vi "Main.vi"() -> ()   [LabVIEW 2016]
uses:
  Experiment States.ctl
  <vilib>/DAQmx/read.llb/DAQmx Read (Analog 2D DBL NChan NSamp).vi
  <vilib>/DAQmx/miscellaneous.llb/DAQmx Fill In Error Info.vi
panel:
  out "T1 12":dbl
  out "T1 11":dbl
  out "T1 10":dbl
  out "T1 9":dbl
  out "T1 8":dbl
  out "T1 7":dbl
  out "T1 6":dbl
  out "T1 5":dbl
  out "T1 4":dbl
  out "T1 3":dbl
  out "T1 2":dbl
  out "T1":dbl
  out "Thermocouple 12":cluster{"X":dbl, "Y":dbl}[](graph)
  out "Thermocouple 11":cluster{"X":dbl, "Y":dbl}[](graph)
  out "Thermocouple 10":cluster{"X":dbl, "Y":dbl}[](graph)
  out "Thermocouple 9":cluster{"X":dbl, "Y":dbl}[](graph)
  out "Thermocouple 8":cluster{"X":dbl, "Y":dbl}[](graph)
  out "Thermocouple 7":cluster{"X":dbl, "Y":dbl}[](graph)
  out "Thermocouple 6":cluster{"X":dbl, "Y":dbl}[](graph)
  out "Thermocouple 5":cluster{"X":dbl, "Y":dbl}[](graph)
  out "Thermocouple 4":cluster{"X":dbl, "Y":dbl}[](graph)
  out "Thermocouple 3":cluster{"X":dbl, "Y":dbl}[](graph)
  out "Thermocouple 2":cluster{"X":dbl, "Y":dbl}[](graph)
  out "Thermocouple 1":cluster{"X":dbl, "Y":dbl}[](graph)
  in  "Thermocouple 12 Channel":tag
  in  "Thermocouple 11 Channel":tag
  in  "Thermocouple 10 Channel":tag
  in  "Thermocouple 9 Channel":tag
  in  "Thermocouple 8 Channel":tag
  in  "Thermocouple 7 Channel":tag
  in  "Thermocouple 6 Channel":tag
  in  "Thermocouple 5 Channel":tag
  in  "Thermocouple 4 Channel":tag
  in  "Thermocouple 3 Channel":tag
  in  "Thermocouple 2 Channel":tag
  in  "Thermocouple 1 Channel":tag
  in  "End Experiment?":bool
  in  "Start":bool
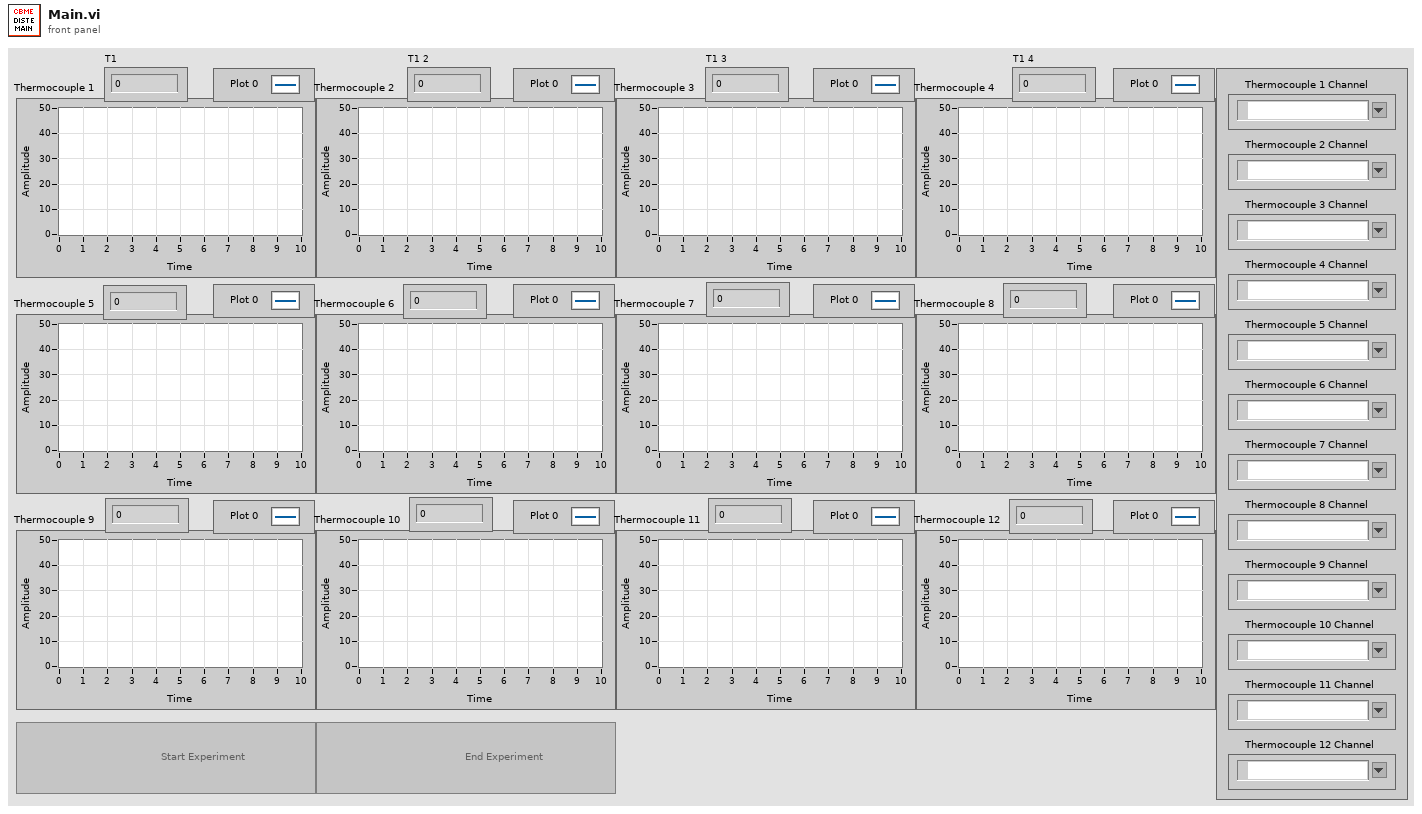
[diagram p1: front panel]
types:
  T1 = typedef "Experiment States.ctl" = enum16{"Setup", "Data Collection", "Export", "Finish"}
  T2 = enum8{"Enabled", "Disabled", "Disabled and Grayed Out"}
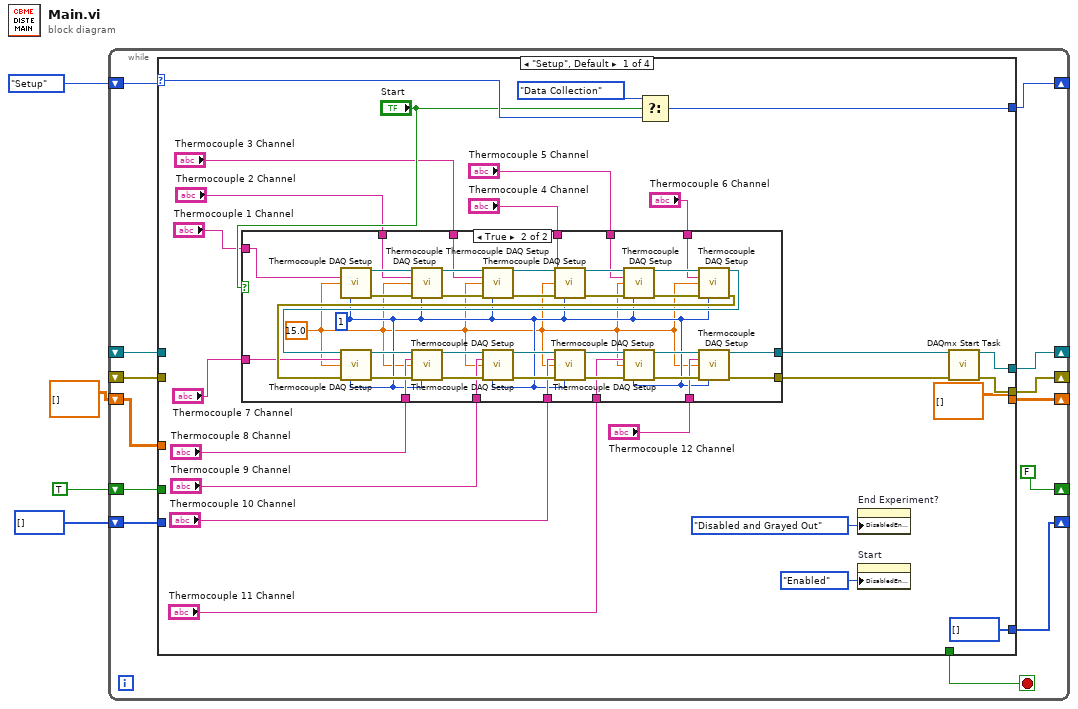
[diagram p0: block diagram]
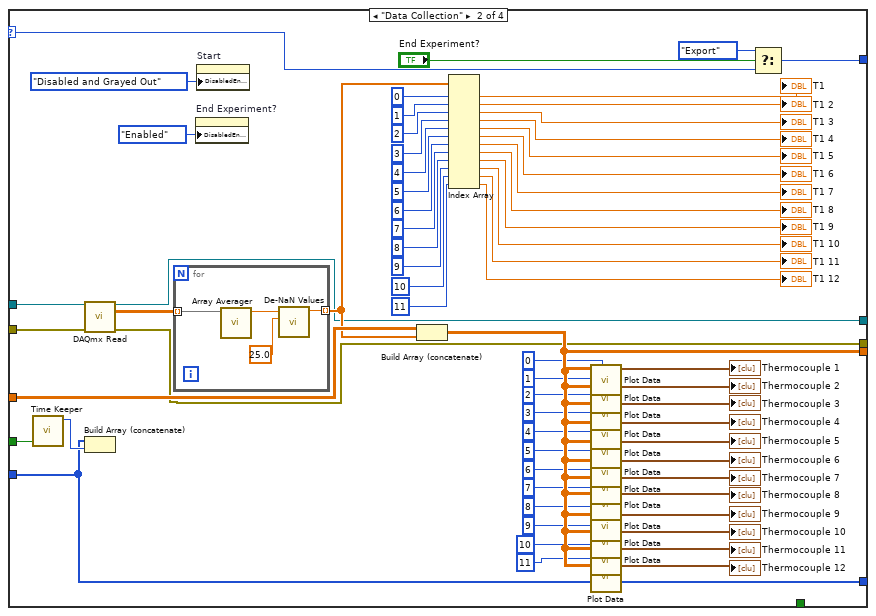
[diagram p3: hidden frame]
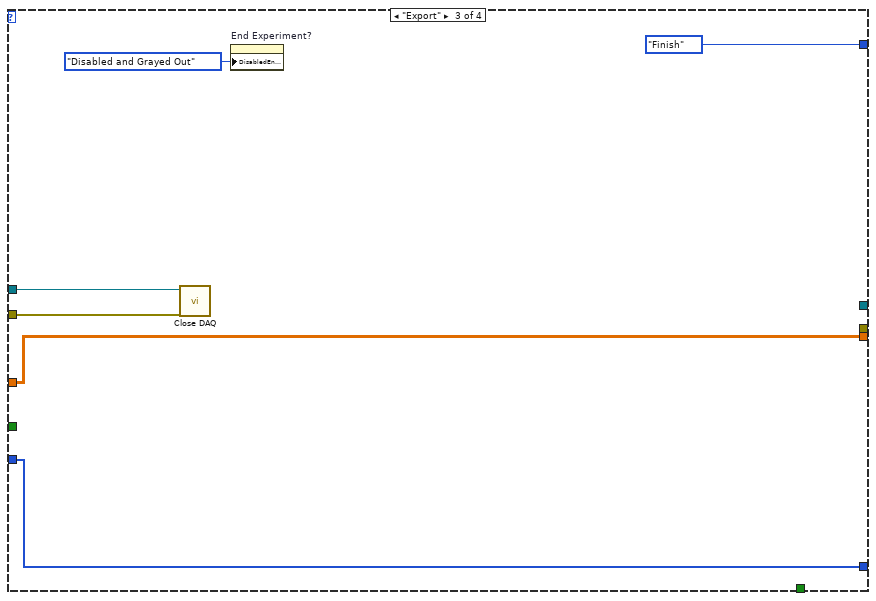
[diagram p4: hidden frame]
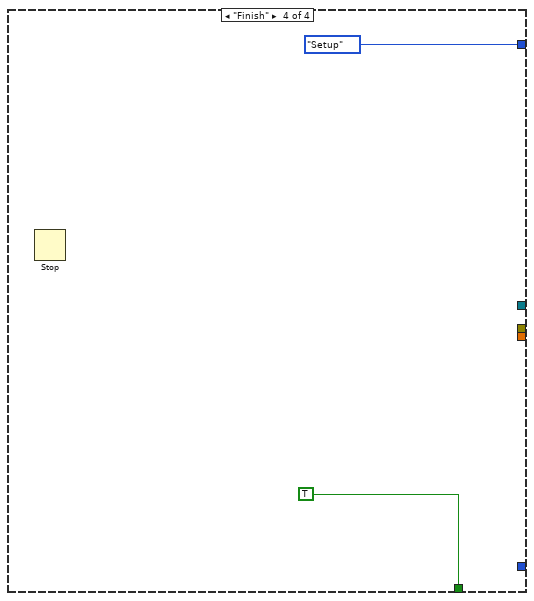
[diagram p5: hidden frame]
diagram:
  n1 = while {
    shift-right: [w16] -> _
    shift-left: Experiment_States."Setup" ("Enum") -> [w17]
    shift-right: [w13] -> _
    shift-left: _ -> [w11]
    shift-right: [w14] -> _
    shift-left: _ -> [w12]
    shift-right: [w10] -> _
    shift-left: dbl[][] [] -> [w9]
    shift-right: [FALSE ("Reset?")] -> _
    shift-left: TRUE ("Reset?") -> [w8]
    shift-right: [w5] -> _
    shift-left: u32[] [] -> [w7]
    stop <- w15 stop-if-true
    n2 = case shown="\"Setup\", Default" w17 {
      selector: w17 -> [w41 w142 _ _]
      tunnel: [w39 w144 Experiment_States."Finish" ("Enum") Experiment_States."Setup" ("Enum")] -> w16
      tunnel: [_ _ _ TRUE] -> w15
      tunnel: [w24 w81 _ _] -> w14
      tunnel: [w22 w80 _ _] -> w13
      tunnel: w12 -> [_ w140 w151 _]
      tunnel: w11 -> [_ w139 w150 _]
      tunnel: [dbl[][] [] w97 w152 _] -> w10
      tunnel: w9 -> [_ w113 w152 _]
      tunnel: w8 -> [_ w110 _ _]
      tunnel: w7 -> [_ w84 w153 _]
      tunnel: [u32[] [] w84 w153 _] -> w5
      frame "Setup", Default {
        n3 = case shown="True" "Start" {
          tunnel: [_ w57] -> w38
          tunnel: [_ w56] -> w23
          tunnel: "Thermocouple 1 Channel" -> [_ w55]
          tunnel: "Thermocouple 2 Channel" -> [_ w54]
          tunnel: "Thermocouple 3 Channel" -> [_ w53]
          tunnel: "Thermocouple 4 Channel" -> [_ w52]
          tunnel: "Thermocouple 5 Channel" -> [_ w51]
          tunnel: "Thermocouple 6 Channel" -> [_ w50]
          tunnel: "Thermocouple 7 Channel" -> [_ w49]
          tunnel: "Thermocouple 8 Channel" -> [_ w48]
          tunnel: "Thermocouple 9 Channel" -> [_ w47]
          tunnel: "Thermocouple 10 Channel" -> [_ w46]
          tunnel: "Thermocouple 11 Channel" -> [_ w45]
          tunnel: "Thermocouple 12 Channel" -> [_ w44]
          frame False {
          }
          frame True {
            w42 = 15.0 ("Sample Rate")
            w43 = 1 ("samples per channel")
            n4 = call "Thermocouple DAQ Setup.vi"("physical channels"=w55, "Sample Rate"=w42, "samples per channel"=w43) -> ("task out"=w63:refnum<k21>, "error out"=w79:errorcluster)  [unwired: 11 in]
            n5 = call "Thermocouple DAQ Setup.vi"("task in"=w63, "physical channels"=w54, "Sample Rate"=w42, "error in"=w79, "samples per channel"=w43) -> ("task out"=w64:refnum<k21>, "error out"=w78:errorcluster)  [unwired: 9 in]
            n6 = call "Thermocouple DAQ Setup.vi"("task in"=w64, "physical channels"=w53, "Sample Rate"=w42, "error in"=w78, "samples per channel"=w43) -> ("task out"=w65:refnum<k21>, "error out"=w77:errorcluster)  [unwired: 9 in]
            n7 = call "Thermocouple DAQ Setup.vi"("task in"=w65, "physical channels"=w52, "Sample Rate"=w42, "error in"=w77, "samples per channel"=w43) -> ("task out"=w66:refnum<k21>, "error out"=w76:errorcluster)  [unwired: 9 in]
            n8 = call "Thermocouple DAQ Setup.vi"("task in"=w66, "physical channels"=w51, "Sample Rate"=w42, "error in"=w76, "samples per channel"=w43) -> ("task out"=w67:refnum<k21>, "error out"=w75:errorcluster)  [unwired: 9 in]
            n9 = call "Thermocouple DAQ Setup.vi"("task in"=w67, "physical channels"=w50, "Sample Rate"=w42, "error in"=w75, "samples per channel"=w43) -> ("task out"=w68:refnum<k21>, "error out"=w69:errorcluster)  [unwired: 9 in]
            n10 = call "Thermocouple DAQ Setup.vi"("task in"=w68, "physical channels"=w49, "Sample Rate"=w42, "error in"=w69, "samples per channel"=w43) -> ("task out"=w62:refnum<k21>, "error out"=w74:errorcluster)  [unwired: 9 in]
            n11 = call "Thermocouple DAQ Setup.vi"("task in"=w62, "physical channels"=w48, "Sample Rate"=w42, "error in"=w74, "samples per channel"=w43) -> ("task out"=w61:refnum<k21>, "error out"=w73:errorcluster)  [unwired: 9 in]
            n12 = call "Thermocouple DAQ Setup.vi"("task in"=w61, "physical channels"=w47, "Sample Rate"=w42, "error in"=w73, "samples per channel"=w43) -> ("task out"=w60:refnum<k21>, "error out"=w72:errorcluster)  [unwired: 9 in]
            n13 = call "Thermocouple DAQ Setup.vi"("task in"=w60, "physical channels"=w46, "Sample Rate"=w42, "error in"=w72, "samples per channel"=w43) -> ("task out"=w59:refnum<k21>, "error out"=w71:errorcluster)  [unwired: 9 in]
            n14 = call "Thermocouple DAQ Setup.vi"("task in"=w59, "physical channels"=w45, "Sample Rate"=w42, "error in"=w71, "samples per channel"=w43) -> ("task out"=w58:refnum<k21>, "error out"=w70:errorcluster)  [unwired: 9 in]
            n15 = call "Thermocouple DAQ Setup.vi"("task in"=w58, "physical channels"=w44, "Sample Rate"=w42, "error in"=w70, "samples per channel"=w43) -> ("task out"=w57:refnum<k21>, "error out"=w56:errorcluster)  [unwired: 9 in]
          }
        }
        n16 = Select(t=Experiment_States."Data Collection", s="Start", f=w41) -> (s? t:f=w39:T1)
        n17 = property on="End Experiment?" class="Bool"("DisabledEnum"=T2."Disabled and Grayed Out" ("Disabled")) -> ()  [unwired: 2 in, 2 out]
        n18 = property on="Start" class="Bool"("DisabledEnum"=T2."Enabled" ("Disabled")) -> ()  [unwired: 2 in, 2 out]
        n19 = call <vilib>:"DAQmx Start Task.vi"("task/channels in"=w38, "error in"=w23) -> ("task out"=w24:refnum<k21>, "error out"=w22:errorcluster)  [unwired: 12 in]
      }
      frame "Data Collection" {
        n20 = call "Time Keeper.vi"("Reset?"=w110) -> ("Time Elapsed (ms)"=w109:u32)  [unwired: 10 in]
        n21 = call-poly <vilib>:"DAQmx Read.vi"("task/channels in"=w140, "error in"=w139) -> ("task out"=w81:refnum<k21>, "data"=w138:dbl[][], "error out"=w80:errorcluster)  [unwired: 11 in]
        n22 = Build Array (concatenate)(w84, w109) -> ()  [unwired: 1 out]
        n23 = for {
          tunnel: w138 -> [w148] mode=indexing
          tunnel: [w145] -> w112 mode=indexing
          n24 = call "Array Averager.vi"("Array"=w148) -> ("Averaged Array"=w147:dbl)  [unwired: 10 in]
          n25 = call "De-NaN Values.vi"("Last Valid"=25.0, "Input"=w147) -> ("De-NaN"=w145:dbl)  [unwired: 9 in]
        }
        n26 = property on="End Experiment?" class="Bool"("DisabledEnum"=T2."Enabled" ("Disabled")) -> ()  [unwired: 2 in, 2 out]
        n27 = property on="Start" class="Bool"("DisabledEnum"=T2."Disabled and Grayed Out" ("Disabled")) -> ()  [unwired: 2 in, 2 out]
        n28 = Build Array (concatenate)(w113, w112) -> (w97:dbl[][])
        n29 = Index Array(array=w112, index #1=0 ("index"), index #2=1 ("index"), index #3=2 ("index"), index #4=3 ("index"), index #5=4 ("index"), index #6=5 ("index"), index #7=6 ("index"), index #8=7 ("index"), index #9=8 ("index"), index #10=9 ("index"), index #11=10 ("index"), index #12=11 ("index")) -> (element #1=→"T1":dbl, element #2=→"T1 2":dbl, element #3=→"T1 3":dbl, element #4=→"T1 4":dbl, element #5=→"T1 5":dbl, element #6=→"T1 6":dbl, element #7=→"T1 7":dbl, element #8=→"T1 8":dbl, element #9=→"T1 9":dbl, element #10=→"T1 10":dbl, element #11=→"T1 11":dbl, element #12=→"T1 12":dbl)
        n30 = call "Plot Data.vi"("Array"=w84, "thermocouple (0 index)"=0, "Array 2"=w97) -> ("Thermocouple 1"=→"Thermocouple 1":cluster{"X":dbl, "Y":dbl}[])  [unwired: 8 in]
        n31 = call "Plot Data.vi"("Array"=w84, "thermocouple (0 index)"=1, "Array 2"=w97) -> ("Thermocouple 1"=→"Thermocouple 2":cluster{"X":dbl, "Y":dbl}[])  [unwired: 8 in]
        n32 = call "Plot Data.vi"("Array"=w84, "thermocouple (0 index)"=2, "Array 2"=w97) -> ("Thermocouple 1"=→"Thermocouple 3":cluster{"X":dbl, "Y":dbl}[])  [unwired: 8 in]
        n33 = call "Plot Data.vi"("Array"=w84, "thermocouple (0 index)"=3, "Array 2"=w97) -> ("Thermocouple 1"=→"Thermocouple 4":cluster{"X":dbl, "Y":dbl}[])  [unwired: 8 in]
        n34 = call "Plot Data.vi"("Array"=w84, "thermocouple (0 index)"=4, "Array 2"=w97) -> ("Thermocouple 1"=→"Thermocouple 5":cluster{"X":dbl, "Y":dbl}[])  [unwired: 8 in]
        n35 = call "Plot Data.vi"("Array"=w84, "thermocouple (0 index)"=5, "Array 2"=w97) -> ("Thermocouple 1"=→"Thermocouple 6":cluster{"X":dbl, "Y":dbl}[])  [unwired: 8 in]
        n36 = call "Plot Data.vi"("Array"=w84, "thermocouple (0 index)"=6, "Array 2"=w97) -> ("Thermocouple 1"=→"Thermocouple 7":cluster{"X":dbl, "Y":dbl}[])  [unwired: 8 in]
        n37 = call "Plot Data.vi"("Array"=w84, "thermocouple (0 index)"=7, "Array 2"=w97) -> ("Thermocouple 1"=→"Thermocouple 8":cluster{"X":dbl, "Y":dbl}[])  [unwired: 8 in]
        n38 = call "Plot Data.vi"("Array"=w84, "thermocouple (0 index)"=8, "Array 2"=w97) -> ("Thermocouple 1"=→"Thermocouple 9":cluster{"X":dbl, "Y":dbl}[])  [unwired: 8 in]
        n39 = call "Plot Data.vi"("Array"=w84, "thermocouple (0 index)"=9, "Array 2"=w97) -> ("Thermocouple 1"=→"Thermocouple 10":cluster{"X":dbl, "Y":dbl}[])  [unwired: 8 in]
        n40 = call "Plot Data.vi"("Array"=w84, "thermocouple (0 index)"=10, "Array 2"=w97) -> ("Thermocouple 1"=→"Thermocouple 11":cluster{"X":dbl, "Y":dbl}[])  [unwired: 8 in]
        n41 = call "Plot Data.vi"("Array"=w84, "thermocouple (0 index)"=11, "Array 2"=w97) -> ("Thermocouple 1"=→"Thermocouple 12":cluster{"X":dbl, "Y":dbl}[])  [unwired: 8 in]
        n42 = Select(t=Experiment_States."Export", s="End Experiment?", f=w142) -> (s? t:f=w144:T1)
      }
      frame "Export" {
        n43 = call "Close DAQ.vi"("error in (no error)"=w150, "Refnum in"=w151) -> ()  [unwired: 10 in]
        n44 = property on="End Experiment?" class="Bool"("DisabledEnum"=T2."Disabled and Grayed Out" ("Disabled")) -> ()  [unwired: 2 in, 2 out]
      }
      frame "Finish" {
        n45 = Stop() -> ()  [unwired: 1 in]
      }
    }
  }
